vi "Fill Out Project Summary.vi"(7 "Project Summary":T1, 8 "error in (no error)":errorcluster, 11 "NI_report in":refnum<class "NI_report.lvclass">) -> (0 "error out":errorcluster, 3 "NI_report out":refnum<class "NI_report.lvclass">)   [LabVIEW 2014]
uses:
  <vilib>/Utility/NIReport.llb/NI_report.lvclass
  Type Defs/TYPE_Project Summary.ctl
  <vilib>/addons/_office/NI_ReportGenerationToolkit.lvlib
  <vilib>/Utility/NIReport.llb/Excel/NI_Excel.lvclass
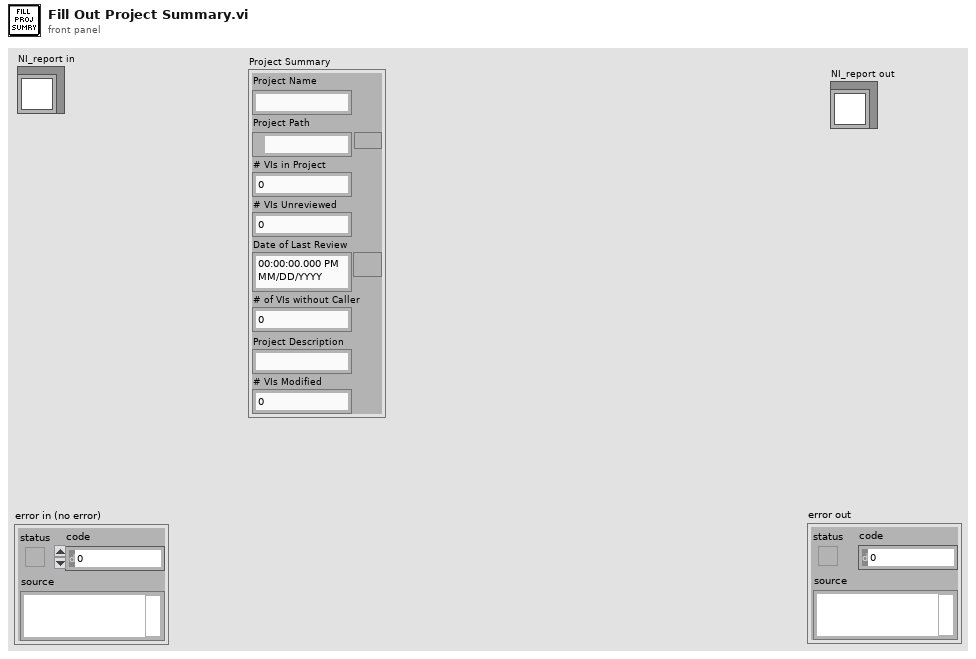
[diagram p1: front panel]
types:
  T1 = typedef "TYPE_Project Summary.ctl" = cluster{"Project Name":string, "Project Path":path, "# VIs in Project":i32, "# VIs Unreviewed":i32, "Date of Last Review":timestamp, "# of VIs without Caller":i32, "Project Description":string, "# VIs Modified":i32}
  T2 = cluster{"on/off":bool, "weight":i32, "color":u32}
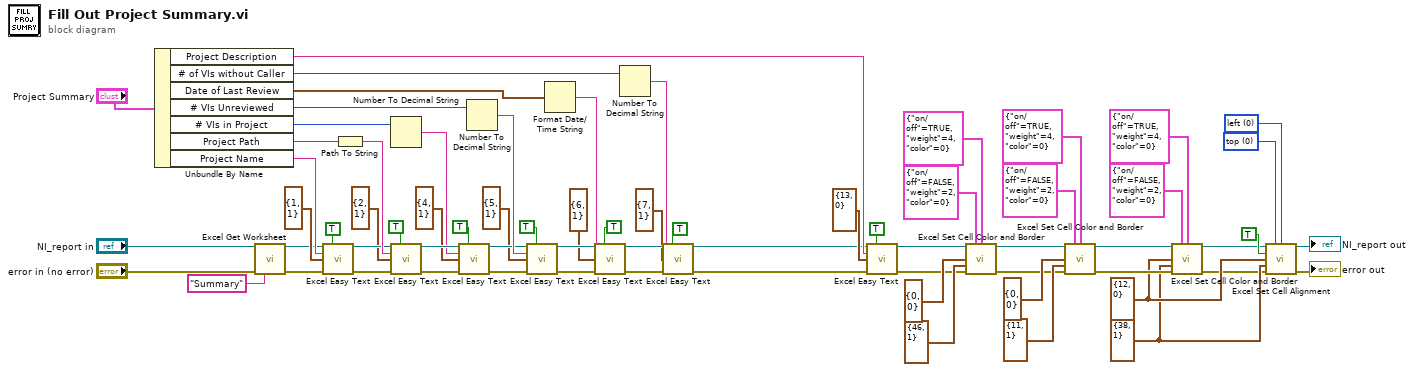
[diagram p0: block diagram]
diagram:
  w3 = cluster{"row":i32, "column":i32} {"row"=38, "column"=1} ("end (-1, -1)")
  w4 = cluster{"row":i32, "column":i32} {"row"=12, "column"=0} ("start (-1, -1)")
  w18 = 0 items=["left", "center", "right"] ("horizontal alignment (left)")
  w19 = 0 items=["top", "center", "bottom"] ("vertical alignment (top)")
  n1 = Unbundle By Name("Project Summary") -> ("Project Description"=w69:string, "# of VIs without Caller"=w64:i32, "Date of Last Review"=w42:timestamp, "# VIs Unreviewed"=w62:i32, "# VIs in Project"=w50:i32, "Project Path"=w38:path, "Project Name"=w33:string)
  n2 = call <vilib>:"Excel Get Worksheet.vi"("report in"="NI_report in", "error in (no error)"="error in (no error)", "name (\"\")"="Summary" ("name (\"\")")) -> ("report out"=w27:refnum<class "NI_report.lvclass">, "error out"=w28:errorcluster)  [unwired: 11 in]
  n3 = call <vilib>:"Excel Easy Text.vi"("report in"=w27, "border? (F)"=TRUE, "text"=w33, "start (-1, -1)"=cluster{"row":i32, "column":i32} {"row"=1, "column"=1}, "error in (no error)"=w28) -> ("report out"=w37:refnum<class "NI_report.lvclass">, "error out"=w36:errorcluster)  [unwired: 6 in, 3 out]
  n4 = Path To String(path=w38) -> (string=w39:string)
  n5 = Number To Decimal String(number=w50) -> (decimal integer string=w51:string)  [unwired: 1 in]
  n6 = call <vilib>:"Excel Easy Text.vi"("report in"=w37, "border? (F)"=TRUE, "text"=w39, "start (-1, -1)"=cluster{"row":i32, "column":i32} {"row"=2, "column"=1}, "error in (no error)"=w36) -> ("report out"=w52:refnum<class "NI_report.lvclass">, "error out"=w53:errorcluster)  [unwired: 6 in, 3 out]
  n7 = call <vilib>:"Excel Easy Text.vi"("report in"=w52, "border? (F)"=TRUE, "text"=w51, "start (-1, -1)"=cluster{"row":i32, "column":i32} {"row"=4, "column"=1}, "error in (no error)"=w53) -> ("report out"=w54:refnum<class "NI_report.lvclass">, "error out"=w55:errorcluster)  [unwired: 6 in, 3 out]
  n8 = Number To Decimal String(number=w62) -> (decimal integer string=w63:string)  [unwired: 1 in]
  n9 = call <vilib>:"Excel Easy Text.vi"("report in"=w54, "border? (F)"=TRUE, "text"=w63, "start (-1, -1)"=cluster{"row":i32, "column":i32} {"row"=5, "column"=1}, "error in (no error)"=w55) -> ("report out"=w56:refnum<class "NI_report.lvclass">, "error out"=w57:errorcluster)  [unwired: 6 in, 3 out]
  n10 = Format Date/Time String(seconds (now)=w42) -> (date/time string=w43:string)  [unwired: 2 in]
  n11 = call <vilib>:"Excel Easy Text.vi"("report in"=w56, "border? (F)"=TRUE, "text"=w43, "start (-1, -1)"=cluster{"row":i32, "column":i32} {"row"=6, "column"=1}, "error in (no error)"=w57) -> ("report out"=w58:refnum<class "NI_report.lvclass">, "error out"=w59:errorcluster)  [unwired: 6 in, 3 out]
  n12 = Number To Decimal String(number=w64) -> (decimal integer string=w65:string)  [unwired: 1 in]
  n13 = call <vilib>:"Excel Easy Text.vi"("report in"=w58, "border? (F)"=TRUE, "text"=w65, "start (-1, -1)"=cluster{"row":i32, "column":i32} {"row"=7, "column"=1}, "error in (no error)"=w59) -> ("report out"=w61:refnum<class "NI_report.lvclass">, "error out"=w60:errorcluster)  [unwired: 6 in, 3 out]
  n14 = call <vilib>:"Excel Easy Text.vi"("report in"=w61, "border? (F)"=TRUE, "text"=w69, "start (-1, -1)"=cluster{"row":i32, "column":i32} {"row"=13, "column"=0}, "error in (no error)"=w60) -> ("report out"=w13:refnum<class "NI_report.lvclass">, "error out"=w12:errorcluster)  [unwired: 6 in, 3 out]
  n15 = call <vilib>:"Excel Set Cell Color and Border.vi"("report in"=w13, "inside border"=T2 {"on/off"=FALSE, "weight"=2, "color"=0}, "outside border"=T2 {"on/off"=TRUE, "weight"=4, "color"=0}, "start (-1, -1)"=cluster{"row":i32, "column":i32} {"row"=0, "column"=0}, "end (-1, -1)"=cluster{"row":i32, "column":i32} {"row"=46, "column"=1}, "error in (no error)"=w12) -> ("report out"=w11:refnum<class "NI_report.lvclass">, "error out"=w10:errorcluster)  [unwired: 8 in]
  n16 = call <vilib>:"Excel Set Cell Color and Border.vi"("report in"=w11, "inside border"=T2 {"on/off"=FALSE, "weight"=2, "color"=0}, "outside border"=T2 {"on/off"=TRUE, "weight"=4, "color"=0}, "start (-1, -1)"=cluster{"row":i32, "column":i32} {"row"=0, "column"=0}, "end (-1, -1)"=cluster{"row":i32, "column":i32} {"row"=11, "column"=1}, "error in (no error)"=w10) -> ("report out"=w6:refnum<class "NI_report.lvclass">, "error out"=w5:errorcluster)  [unwired: 8 in]
  n17 = call <vilib>:"Excel Set Cell Color and Border.vi"("report in"=w6, "inside border"=T2 {"on/off"=FALSE, "weight"=2, "color"=0}, "outside border"=T2 {"on/off"=TRUE, "weight"=4, "color"=0}, "start (-1, -1)"=w4, "end (-1, -1)"=w3, "error in (no error)"=w5) -> ("report out"=w1:refnum<class "NI_report.lvclass">, "error out"=w2:errorcluster)  [unwired: 8 in]
  n18 = call <vilib>:"Excel Set Cell Alignment.vi"("report in"=w1, "vertical alignment (top)"=w19, "horizontal alignment (left)"=w18, "wrap text? (F)"=TRUE, "start (-1, -1)"=w4, "end (-1, -1)"=w3, "error in (no error)"=w2) -> ("report out"=→"NI_report out":refnum<class "NI_report.lvclass">, "error out"=→"error out":errorcluster)  [unwired: 7 in]
